vi "AlliGator Global Fit Decay Pre-conditioning.vi"(0 "XYGraph in":refnum<vi>, 5 "Selected Plots":i32[](array[numeric]), 7 "Max Decay Percentile (1)":dbl=1.0, 9 "Min Decay Percentile (0)":dbl, 11 "error in (no error)":errorcluster) -> (2 "Index Max Array":i32[](array[numeric]), 3 "Valid Plot Indices":i32[](array[numeric]), 4 "XYGraph out":refnum<vi>, 6 "Full Decays":cluster{"t Array":dbl[], "Value Array":dbl[]}[](array[cluster]), 8 "Clipped Decays":cluster{"t Array":dbl[], "Value Array":dbl[]}[](array[cluster]), 10 "Plot Names":string[](array[string]), 12 "Message":string, 13 "Is Valid?":bool, 14 "# Points":i32[](array[numeric]), 15 "error out":errorcluster)   [LabVIEW 2021, in "AlliGator Global Decay Fit.lvlib"]
uses:
  AlliGator Global Decay Fit.lvlib
  5b90b548-0d44-4b42-95e1-3915b01d176a.vi
  Decay Fit/AlliGator Decay Fit.lvlib
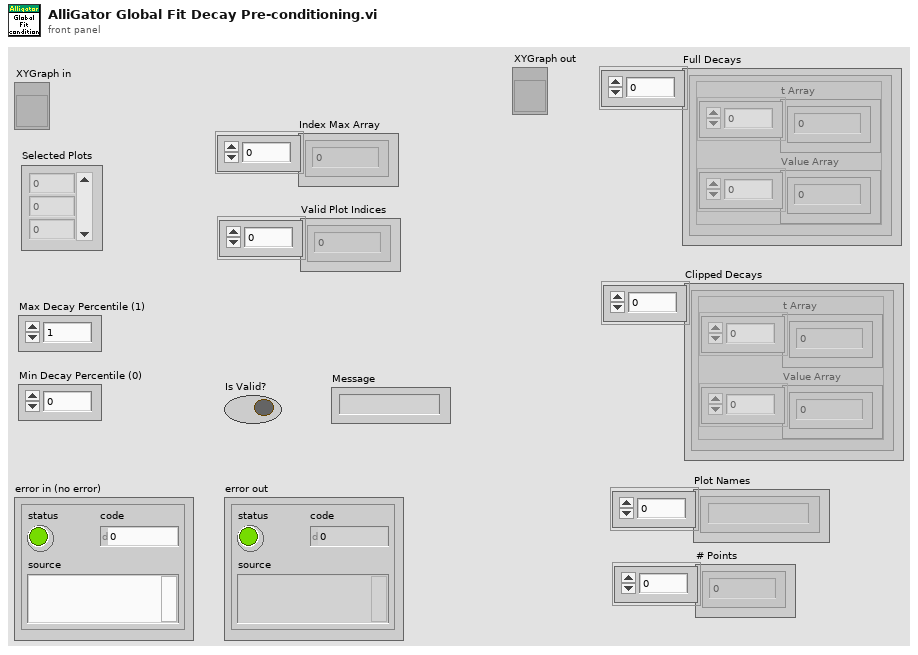
[diagram p1: front panel]
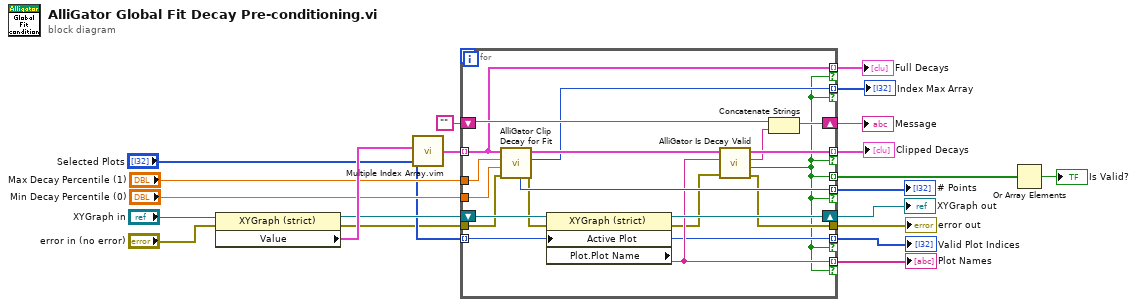
[diagram p0: block diagram]
diagram:
  n1 = property class="XYGraph (strict)"(reference="XYGraph in", error in="error in (no error)") -> (reference out=w15:refnum<vi>, error out=w13:errorcluster, "Value"=w19:cluster{"X Array":dbl[], "Y Array":dbl[]}[])
  n2 = call "Multiple Index Array.vim"("Index Array"="Selected Plots", "Array"=w19) -> ("Selected Element(s)"=w18:cluster{"X Array":dbl[], "Y Array":dbl[]}[])  [unwired: 4 in]
  n3 = for {
    tunnel: w18 -> [w24] mode=indexing
    tunnel: "Max Decay Percentile (1)" -> [w40]
    tunnel: "Min Decay Percentile (0)" -> [w39]
    tunnel: [w37] -> w2 mode=indexing if=w22
    tunnel: [w36] -> w9 mode=indexing if=w22
    shift-right: [w32] -> w10
    shift-left: "" -> [w31]
    shift-right: [w34] -> w11
    shift-left: w15 -> [w35]
    tunnel: "Selected Plots" -> [w29] mode=indexing
    tunnel: [w30] -> w8 mode=indexing if=w22
    tunnel: [w29] -> w4 mode=indexing if=w22
    tunnel: [w22] -> w7 mode=indexing
    tunnel: w13 -> [w27]
    tunnel: [w25] -> w5
    tunnel: [w24] -> w3 mode=indexing if=w22
    tunnel: [w23] -> w1 mode=indexing if=w22
    n4 = call "AlliGator Clip Decay for Fit.vi"("Error In"=w27, "Min Decay Percentile (0)"=w39, "Max Decay Percentile (1)"=w40, "Decay in"=w24) -> ("Error Out"=w28:errorcluster, "Index Max"=w23:i32, "Clipped Decay out"=w38:cluster{"t Array":dbl[], "Value Array":dbl[]}, "# Points"=w37:i32)  [unwired: 3 in, 1 out]
    n5 = property class="XYGraph (strict)"(reference=w35, error in=w28, "Active Plot"=w29) -> (reference out=w34:refnum<vi>, error out=w26:errorcluster, "Plot.Plot Name"=w30:string)
    n6 = call "AlliGator Is Decay Valid.vi"("Error In"=w26, "Plot Name"=w30, "Decay"=w38) -> ("Error Out"=w25:errorcluster, "Is Valid?"=w22:bool, "Message"=w33:string, "Decay (dup)"=w36:cluster{"t Array":dbl[], "Value Array":dbl[]})  [unwired: 5 in]
    n7 = Concatenate Strings(w31, w33) -> (w32:string)
  }
  "Plot Names" <- w8
  "Message" <- w10
  "error out" <- w5
  "Clipped Decays" <- w9
  "# Points" <- w2
  "XYGraph out" <- w11
  "Valid Plot Indices" <- w4
  "Full Decays" <- w3
  "Index Max Array" <- w1
  n8 = Or Array Elements(Boolean array=w7) -> (logical OR=→"Is Valid?":bool)
